vi "Get Current Users Groups.vi"(8 "error in (no error)":errorcluster) -> (0 "error out":errorcluster, 3 "groups":string[](array[string]))   [LabVIEW 2017, in "Windows Security.lvlib"]
doc: "Returns the current (logged in) user's groups."
uses:
  System.DirectoryServices.AccountManagement
  Windows Security.lvlib
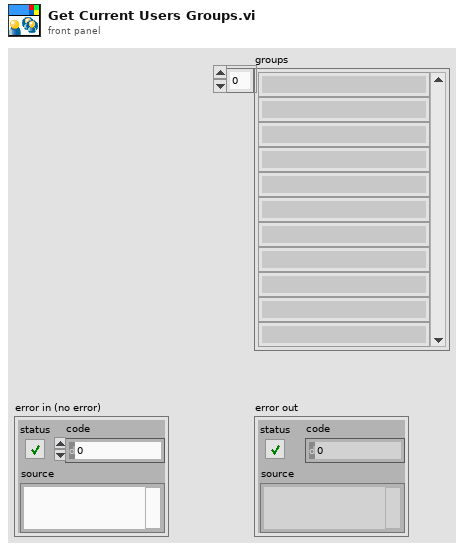
[diagram p1: front panel]
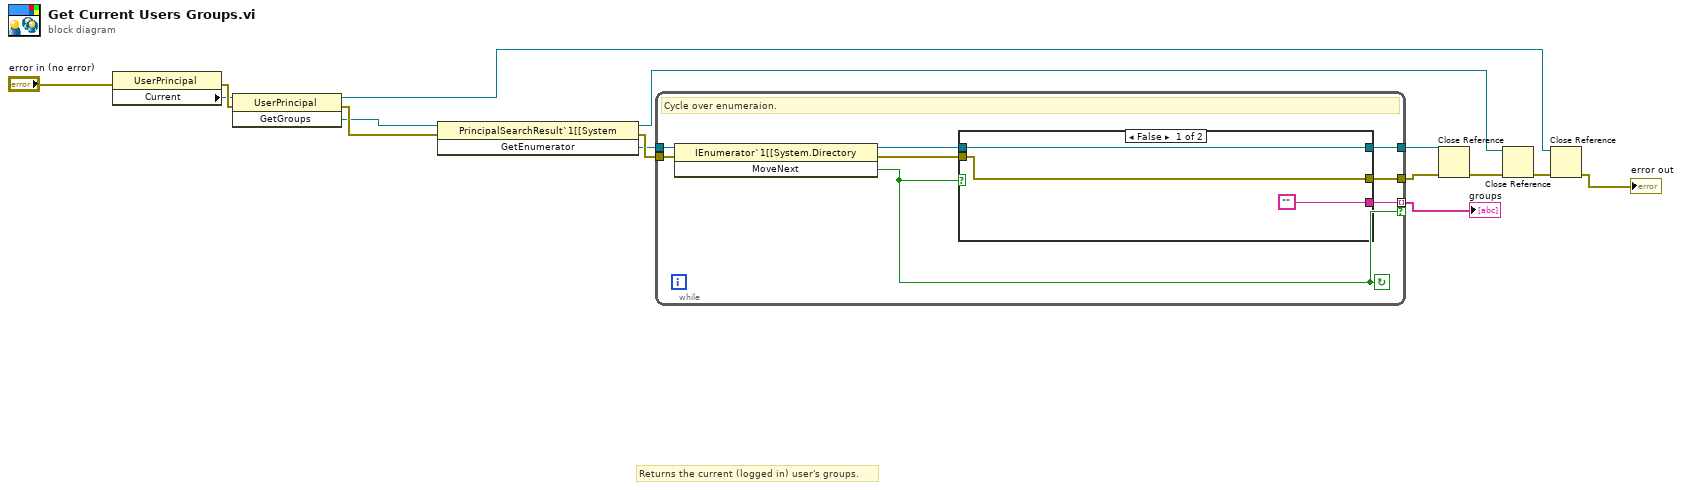
[diagram p0: block diagram]
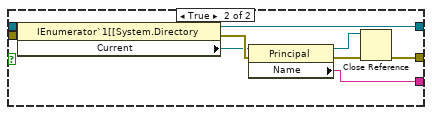
[diagram p2: hidden frame]
diagram:
  # "Returns the current (logged in) user's groups."
  n1 = property class="UserPrincipal"(error in="error in (no error)") -> (error out=w13:errorcluster, "Current"=w10:refnum<k24>)  [unwired: 1 in, 1 out]
  n2 = invoke class="UserPrincipal" method="GetGroups"(reference=w10, error in=w13) -> (reference out=w1:refnum<k24>, error out=w14:errorcluster, "rvices.AccountManagement, Version=0.0.0.0, Culture=neutral, PublicKeyToken=b77a5c561934e089\tGetGroups"=w12:refnum<k24>)  [unwired: 1 in]
  n3 = invoke class="PrincipalSearchResult`1[[System" method="GetEnumerator"(reference=w12, error in=w14) -> (reference out=w2:refnum<k24>, error out=w15:errorcluster, "GetEnumerator"=w11:refnum<k24>)  [unwired: 1 in]
  n4 = while {
    tunnel: w11 -> [w23]
    tunnel: [w21] -> w8 mode=indexing if=w17
    tunnel: w15 -> [w20]
    tunnel: [w18] -> w7
    tunnel: [w16] -> w3
    stop <- w17 continue-if-true
    # "Cycle over enumeraion."
    n5 = invoke class="IEnumerator`1[[System.Directory" method="MoveNext"(reference=w23, error in=w20) -> (reference out=w22:refnum<k24>, error out=w19:errorcluster, "MoveNext"=w17:bool)  [unwired: 1 in]
    n6 = case shown="False" w17 {
      tunnel: w22 -> [w24 w33]
      tunnel: ["" w32] -> w21
      tunnel: w19 -> [w26 w31]
      tunnel: [w26 w28] -> w18
      tunnel: [w24 w27] -> w16
      frame False {
      }
      frame True {
        n7 = property class="IEnumerator`1[[System.Directory"(reference=w33, error in=w31) -> (reference out=w27:refnum<k24>, error out=w35:errorcluster, "Current"=w34:refnum<k24>)
        n8 = property class="Principal"(reference=w34, error in=w35) -> (reference out=w29:refnum<k24>, error out=w30:errorcluster, "Name"=w32:string)
        n9 = Close Reference(reference=w29, error in (no error)=w30) -> (error out=w28:errorcluster)
      }
    }
  }
  "groups" <- w8
  n10 = Close Reference(reference=w3, error in (no error)=w7) -> (error out=w5:errorcluster)
  n11 = Close Reference(reference=w2, error in (no error)=w5) -> (error out=w6:errorcluster)
  n12 = Close Reference(reference=w1, error in (no error)=w6) -> (error out=→"error out":errorcluster)
